vi "Paste Template Code and Wire Error Wires.vi"(8 "error in (no error)":errorcluster, 10 "Position":T1, 11 "DVR API Path":path) -> (0 "error out":errorcluster)   [LabVIEW 2016, in "SLL Class DVR API Generator.lvlib"]
uses:
  SLL Class DVR API Generator.lvlib
  <vilib>/Utility/miscctls.llb/LVPositionTypeDef.ctl
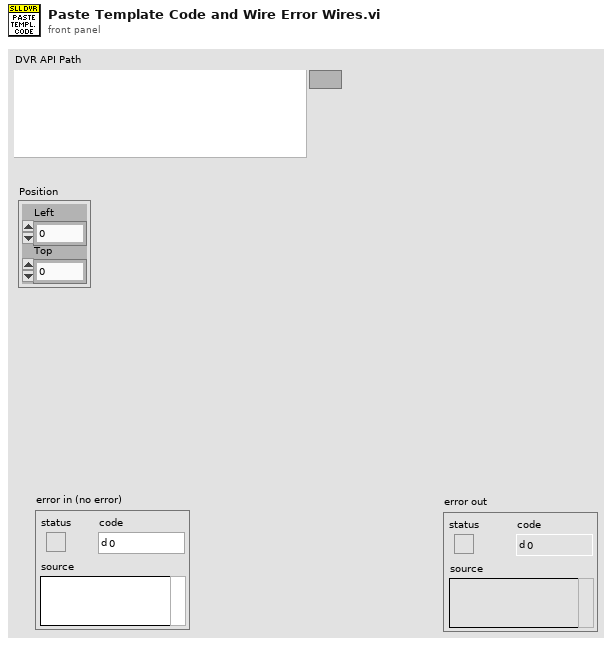
[diagram p1: front panel]
types:
  T1 = typedef "LVPositionTypeDef.ctl" = cluster{"Left":i32, "Top":i32}
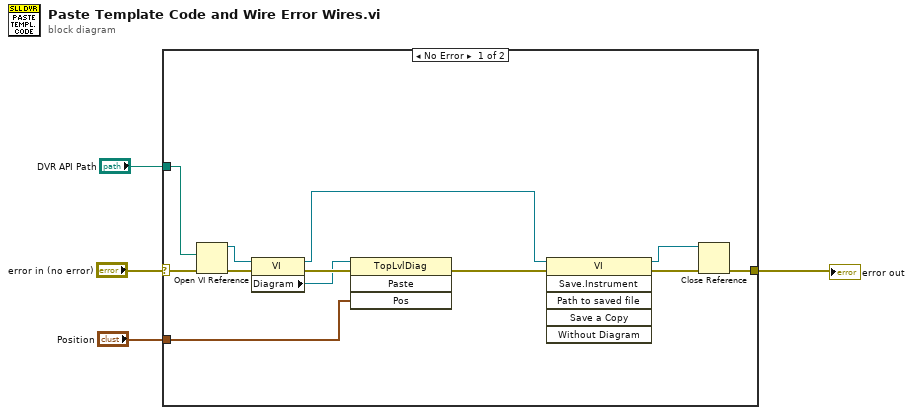
[diagram p0: block diagram]
diagram:
  n1 = case shown="No Error" "error in (no error)" {
    selector: "error in (no error)" -> [w13 w17]
    tunnel: [w7 w17] -> w3
    tunnel: "DVR API Path" -> [w12 _]
    tunnel: "Position" -> [w5 _]
    frame No Error {
      n2 = Open VI Reference(vi path=w12, error in (no error)=w13) -> (vi reference=w10:refnum<vi>, error out=w11:errorcluster)  [unwired: 4 in]
      n3 = property class="VI"(reference=w10, error in=w11) -> (reference out=w8:refnum<vi>, error out=w16:errorcluster, "Diagram"=w15:refnum<vi>)
      n4 = invoke class="TopLvlDiag" method="Paste"(reference=w15, error in=w16, "Pos"=w5) -> (error out=w14:errorcluster)  [unwired: 1 in, 3 out]
      n5 = invoke class="VI" method="Save.Instrument"(reference=w8, error in=w14) -> (reference out=w6:refnum<vi>, error out=w9:errorcluster)  [unwired: 4 in, 4 out]
      n6 = Close Reference(reference=w6, error in (no error)=w9) -> (error out=w7:errorcluster)
    }
    frame Error {
    }
  }
  "error out" <- w3
